vi "Actor Core.vi"(8 "error in":errorcluster, 11 "Network Endpoint":refnum<class "Network Endpoint.lvclass">) -> (0 "error out":errorcluster, 3 "Actor out":refnum<class "Actor.lvclass">)   [LabVIEW 2020, in "Network Endpoint.lvlib" / "Network Endpoint.lvclass"]
doc: "Manages the reader network stream. Waits for a remote writer to connect. Once a connection is established, forwards received messages to its parent node."
uses:
  Network Endpoint.lvclass
  <vilib>/ActorFramework/Actor/Actor.lvclass
  <vilib>/ActorFramework/Message Enqueuer/Message Enqueuer.lvclass
  <vilib>/ActorFramework/Report Error Msg/Report Error Msg.lvclass
  Abstract Classes/Message Stream/Message Stream.lvclass
  <resource>/AFDebug/AF Debug.lvlib
  C:/Program Files (x86)/National Instruments/LabVIEW 2021/vi.lib/ActorFramework/Actor/Actor.lvclass
  C:/Users/allen/Desktop/Network Endpoints with Tests Folder/justACS/network-endpoints/4.0/Source/Network Endpoint/Network Endpoint/Network Endpoint.lvclass
  <vilib>/ActorFramework/Message/Message.lvclass
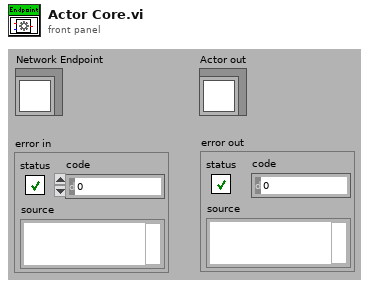
[diagram p1: front panel]
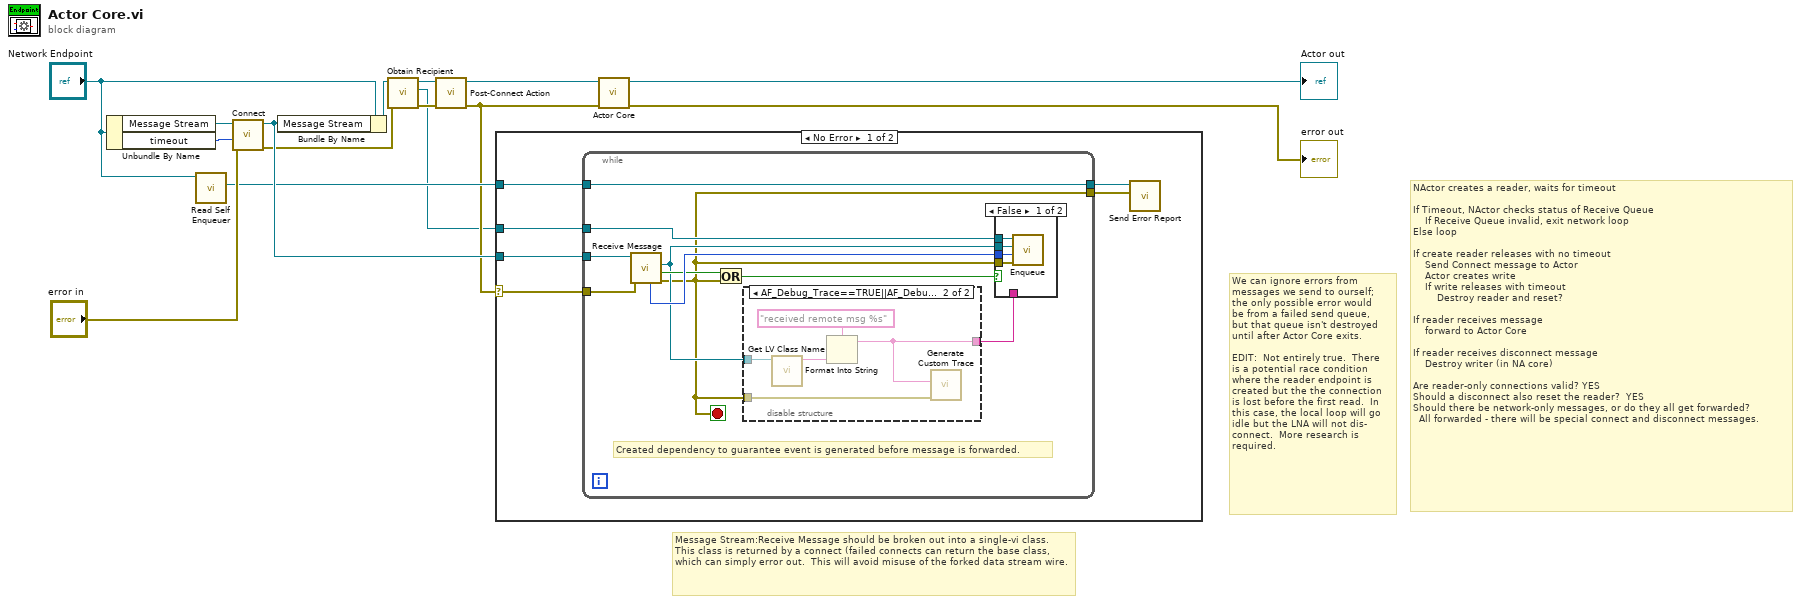
[diagram p0: block diagram]
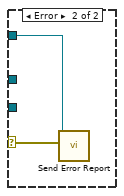
[diagram p4: hidden frame]
diagram:
  # "Message Stream:Receive Message should be broken out into a single-vi class.\nThis class is returned by a connect (failed connects can return the base class, which can simply error out.  This will avoid misuse of the forked data stream wire."
  # "We can ignore errors from\nmessages we send to ourself;\nthe only possible error would\nbe from a failed send queue,\nbut that queue isn't destroyed\nuntil after Actor Core exits.\n\nEDIT:  Not entirely true.  There\nis a potential race condition \nwhere the reader endpoint is\ncreated but the the connection\nis lost before the first read.  In\nthis case, the local loop will go\nidle but the LNA will not dis-\nconnect.  More research is\nrequired."
  # "NActor creates a reader, waits for timeout\n\nIf Timeout, NActor checks status of Receive Queue\n    If Receive Queue invalid, exit network loop\nElse loop\n\nIf create reader releases with no timeout\n    Send Connect message to Actor\n    Actor creates write\n    If write releases with timeout\n        Destroy reader and reset?\n\nIf reader receives message\n    forward to Actor Core\n\nIf reader receives disconnect message\n    Destroy writer (in NA core)\n\nAre reader-only connections valid? YES\nShould a disconnect also reset the reader?  YES\nShould there be network-only messages, or do they all get forwarded?\n  All forwarded - there will be special connect and disconnect messages."
  n1 = Unbundle By Name("Network Endpoint") -> ("Message Stream"=w13:refnum<class "Message Stream.lvclass">, "timeout"=w12:i32)
  n2 = call <vilib>:"Read Self Enqueuer.vi"("Actor"="Network Endpoint") -> ("Self Enqueuer"=w9:refnum<class "Message Enqueuer.lvclass">)  [unwired: 10 in]
  n3 = call-dynamic "Connect.vi"("error in (no error)"="error in", "timeout"=w12, "Message Stream in"=w13) -> ("error out"=w3:errorcluster, "Message Stream out"=w11:refnum<class "Message Stream.lvclass">)  [unwired: 7 in]
  n4 = Bundle By Name(cluster="Network Endpoint", "Message Stream"=w11) -> (w4:refnum<class "Network Endpoint.lvclass">)
  n5 = call-dynamic "Obtain Recipient.vi"("error in (no error)"=w3, "Network Endpoint in"=w4) -> ("error out"=w7:errorcluster, "Recipient Enqueuer"=w1:refnum<class "Message Enqueuer.lvclass">, "Network Endpoint out"=w6:refnum<class "Network Endpoint.lvclass">)  [unwired: 7 in]
  n6 = call-dynamic "Post-Connect Action.vi"("error in (no error)"=w7, "Network Endpoint in"=w6) -> ("error out"=w2:errorcluster, "Network Endpoint out"=w5:refnum<class "Network Endpoint.lvclass">)  [unwired: 8 in]
  n7 = case shown="No Error" w2 {
    selector: w2 -> [w21 w42]
    tunnel: w1 -> [w20 _]
    tunnel: w11 -> [w19 _]
    tunnel: w9 -> [w18 w41]
    frame No Error {
      n8 = while {
        tunnel: w21 -> [w30]
        tunnel: w19 -> [w29]
        tunnel: w20 -> [w31]
        tunnel: [w27] -> w17
        tunnel: w18 -> [w27]
        tunnel: [w22] -> w16
        stop <- w22 stop-if-true
        # "Created dependency to guarantee event is generated before message is forwarded."
        n9 = call-dynamic "Receive Message.vi"("error in (no error)"=w30, "Message Stream in"=w29) -> ("error out"=w22:errorcluster, "Timed out?"=w26:bool, "Message"=w24:refnum<class "Message.lvclass">, "priority"=w28:i32)  [unwired: 5 in, 1 out]
        n10 = Or(x=w26, y=w22) -> (x .or. y?=w25:bool)
        n11 = disable-structure shown="AF_Debug_Trace==TRUE||AF_Debug_Trace==True" {
          disable-tunnel: w22 -> [_ w40]
          disable-tunnel: w24 -> [_ w37]
          disable-tunnel: [_ w36] -> w23
          frame condition #0 (active) {
          }
          frame condition #1 {
            n12 = call <vilib>:"Get LV Class Name.vi"("object"=w37) -> ("class name"=w38:string)  [unwired: 9 in, 1 out]
            n13 = Format Into String(format string="received remote msg %s", w38) -> (resulting string=w36:string)  [unwired: 2 in, 1 out]
            n14 = call <resource>:"Generate Custom Trace.vi"("error in (no error)"=w40, "Custom Action"=w36) -> ()  [unwired: 10 in]
          }
        }
        n15 = case shown="False" w25 {
          tunnel: w31 -> [w35 _]
          tunnel: w24 -> [w34 _]
          tunnel: w28 -> [w33 _]
          tunnel: w22 -> [w32 _]
          tunnel: w23 -> [_ _]
          frame False {
            n16 = call <vilib>:"Enqueue.vi"("error in (no error)"=w32, "Message Priority (Normal)"=w33, "Message"=w34, "Message Enqueuer in"=w35) -> ()  [unwired: 6 in, 2 out]
          }
          frame True {
          }
        }
      }
      n17 = call <vilib>:"Send Error Report.vi"("Error From Sender"=w16, "Message Enqueuer"=w17) -> ()  [unwired: 9 in, 1 out]
    }
    frame Error {
      n18 = call <vilib>:"Send Error Report.vi"("Error From Sender"=w42, "Message Enqueuer"=w41) -> ()  [unwired: 9 in, 1 out]
    }
  }
  n19 = call-parent "Actor Core.vi"("error in"=w2, "Actor in"=w5) -> ("error out"=→"error out":errorcluster, "Actor out"=→"Actor out":refnum<class "Actor.lvclass">)  [unwired: 8 in]
